vi "configureTimingNow.vi"(8 "error in (no error)":errorcluster, 11 "DIO64Output in":refnum<class "DIO64Output.lvclass">) -> (0 "error out":errorcluster, 3 "DIO64Output out":refnum<class "DIO64Output.lvclass">)   [LabVIEW 2009, in "Hardware.lvlib" / "Channels.lvlib" / "DIO64Output.lvclass"]
uses:
  DIO64Output.lvclass
  DIO64Output.lvclass/DIO64Output.ctl
  <userlib>/dio64_32.LLB/DIO64 attribute value.ctl
  <userlib>/dio64_32.LLB/DIO64 attribute id.ctl
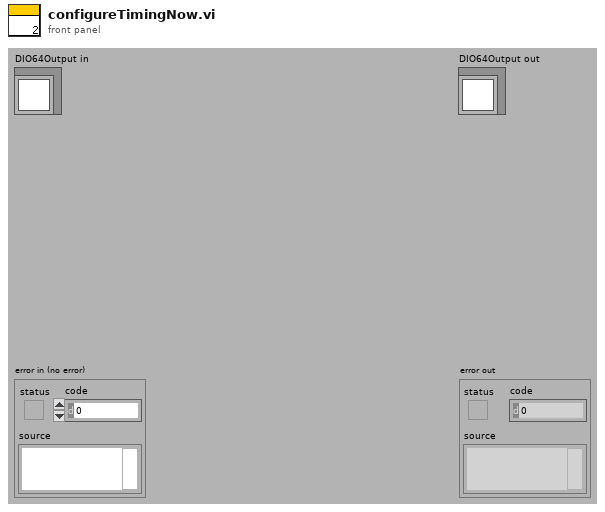
[diagram p1: front panel]
types:
  T1 = cluster{"Master Clock source":string, "Master Clock rate":dbl, "Start trigger line":string, "Scan rate":dbl, "Stop trigger line":string, "Sample Number":dbl}
  T2 = typedef "DIO64 Out Config Control.ctl" = cluster{"flags":enum16{"unused"}, "clock control":T3, "start trigger":T4, "stop trigger":T5, "DAQ clock modulo":u32, "repetitions":u32, "#transitions":u16}
  T3 = typedef "DIO64 clock control.ctl" = enum16{"internal", "external", "trig 0", "OCXO"}
  T4 = typedef "DIO64 start trig.ctl" = cluster{"source":enum16{"none", "internal", "external", "trig 2", "PXI Star"}, "type":enum16{"level", "edge", "edge to edge"}, "sense":enum16{"rising", "falling"}}
  T5 = typedef "DIO64 stop trig.ctl" = cluster{"source":enum16{"none", "internal", "external", "trig 3 in", "output FIFO"}, "type":enum16{"level", "edge"}, "sense":enum16{"falling", "rising"}}
  T6 = typedef "DIO64 attribute value.ctl" = enum16{"default", "long value", "polled", "interrupt", "packet", "demand", "local clock", "external clock", "rtsi/pxi clock", "precision clock", "20MHz", "10MHz", "precision OCXO", "enable", "disable"}
  T7 = typedef "DIO64 attribute id.ctl" = enum16{"input mode", "output mode", "input buffer size", "output buffer size", "major clock source", "input threshold percent", "output threshold percent", "input dma timeout", "rtsi/pxi global enable", "rtsi/pxi clock source", "rtsi clock/pxi trig 7 enable", "external clock enable", "pxi clock enable", "scan clock trig 0 enable", "start trig trig 2 enable", "stop trig trig 3 enable", "daq modulo trig 4 enable", "pxi star enable", "port routing", "staticOutputPorts", "serial number", "rearm enable", "SCLK enable", "FPGA info"}
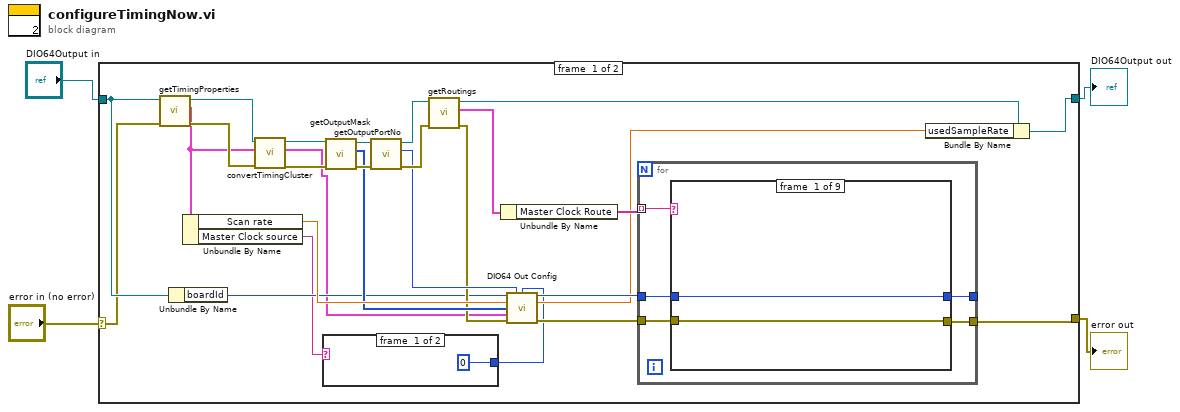
[diagram p0: block diagram]
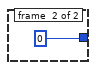
[diagram p2: hidden frame]
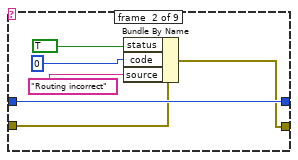
[diagram p3: hidden frame]
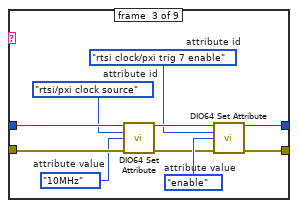
[diagram p4: hidden frame]
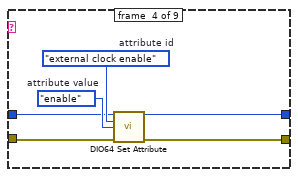
[diagram p5: hidden frame]
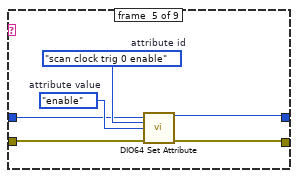
[diagram p6: hidden frame]
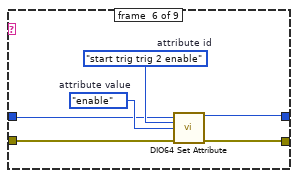
[diagram p7: hidden frame]
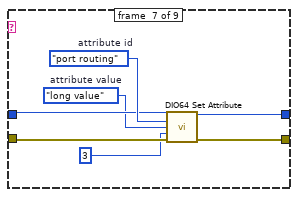
[diagram p8: hidden frame]
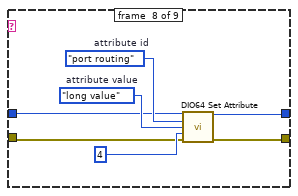
[diagram p9: hidden frame]
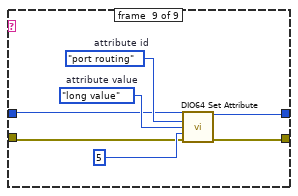
[diagram p10: hidden frame]
diagram:
  n1 = case shown="No Error" "error in (no error)" {
    selector: "error in (no error)" -> [w8 w96]
    tunnel: "DIO64Output in" -> [w10 w97]
    tunnel: [w12 w97] -> w2
    tunnel: [w22 w96] -> w1
    frame #0 {
      n2 = call-dynamic "getTimingProperties.vi"("error in (no error)"=w8, "DigitalOutput.lvclass in"=w10) -> ("error out"=w30:errorcluster, "Timing"=w17:T1, "DigitalOutput.lvclass out"=w31:refnum<class "DIO64Output.lvclass">)  [unwired: 7 in]
      n3 = Unbundle By Name(w10) -> ("boardId"=w9:i32)
      n4 = Unbundle By Name(w17) -> ("Scan rate"=w23:dbl, "Master Clock source"=w7:string)
      n5 = call "convertTimingCluster.vi"("error in (no error)"=w30, "Timing"=w17, "DIO64Output in"=w31) -> ("error out"=w26:errorcluster, "Out Config Control"=w5:T2, "DIO64Output out"=w27:refnum<class "DIO64Output.lvclass">)  [unwired: 6 in]
      n6 = case shown="\"PXI_Trig_00\"" w7 {
        tunnel: [u32 0 ("divider") 0] -> w6
        frame #0 {
        }
        frame #1 {
        }
      }
      n7 = call "getOutputMask.vi"("error in (no error)"=w26, "DIO64Output.lvclass in"=w27) -> ("error out"=w28:errorcluster, "mask"=w18:u16[], "DIO64Output.lvclass out"=w29:refnum<class "DIO64Output.lvclass">)  [unwired: 7 in]
      n8 = call "getOutputPortNo.vi"("error in (no error)"=w28, "DIO64Output.lvclass in"=w29) -> ("error out"=w24:errorcluster, "#ports"=w19:u8, "DIO64Output.lvclass out"=w25:refnum<class "DIO64Output.lvclass">)  [unwired: 7 in]
      n9 = call-dynamic "getRoutings.vi"("error in (no error)"=w24, "DigitalOutput.lvclass in"=w25) -> ("error out"=w14:errorcluster, "Routings"=w21:cluster{"Master Clock Route":string[]}, "DigitalOutput.lvclass out"=w13:refnum<class "DIO64Output.lvclass">)  [unwired: 7 in]
      n10 = Unbundle By Name(w21) -> ("Master Clock Route"=w20:string[])
      n11 = call <userlib>:"DIO64 Out Config.vi"("board in"=w9, "#ports"=w19, "divider"=w6, "scan rate (Hz)"=w23, "mask"=w18, "Config Control"=w5, "error in (no error)"=w14) -> ("board out"=w16:u16, "actual scan rate (Hz)"=w11:dbl, "error out"=w15:errorcluster)  [unwired: 6 in]
      n12 = for {
        tunnel: [w38] -> w22
        tunnel: w15 -> [w37]
        tunnel: w16 -> [w36]
        tunnel: [w35] -> _
        tunnel: w20 -> [w34] mode=indexing
        n13 = case shown="\"Dio64_10MHz to PXI_Trig_07\"" w34 {
          tunnel: [w39 w44 w47 w58 w63 w69 w78 w82 w90] -> w38
          tunnel: w37 -> [w39 w45 w55 w59 w65 w71 w79 w84 w91]
          tunnel: w36 -> [w40 w46 w56 w60 w66 w72 w80 w85 w92]
          tunnel: [w40 w46 w48 w57 w64 w70 w77 w83 w89] -> w35
          frame #0 {
          }
          frame #1 {
            n14 = Bundle By Name(cluster=w45, "status"=TRUE, "code"=0, "source"="Routing incorrect") -> (w44:errorcluster)
          }
          frame #2 {
            w50 = DIO64_attribute_value."enable"  # attribute value
            w51 = DIO64_attribute_id."rtsi clock/pxi trig 7 enable"  # attribute id
            w53 = DIO64_attribute_value."10MHz"  # attribute value
            w54 = DIO64_attribute_id."rtsi/pxi clock source"  # attribute id
            n15 = call <userlib>:"DIO64 Set Attribute.vi"("board in"=w56, "attribute id"=w54, "attribute value"=w53, "error in (no error)"=w55) -> ("board out"=w52:u16, "error out"=w49:errorcluster)  [unwired: 10 in]
            n16 = call <userlib>:"DIO64 Set Attribute.vi"("board in"=w52, "attribute id"=w51, "attribute value"=w50, "error in (no error)"=w49) -> ("board out"=w48:u16, "error out"=w47:errorcluster)  [unwired: 10 in]
          }
          frame #3 {
            w61 = DIO64_attribute_value."enable"  # attribute value
            w62 = DIO64_attribute_id."external clock enable"  # attribute id
            n17 = call <userlib>:"DIO64 Set Attribute.vi"("board in"=w60, "attribute id"=w62, "attribute value"=w61, "error in (no error)"=w59) -> ("board out"=w57:u16, "error out"=w58:errorcluster)  [unwired: 10 in]
          }
          frame #4 {
            w67 = DIO64_attribute_value."enable"  # attribute value
            w68 = DIO64_attribute_id."scan clock trig 0 enable"  # attribute id
            n18 = call <userlib>:"DIO64 Set Attribute.vi"("board in"=w66, "attribute id"=w68, "attribute value"=w67, "error in (no error)"=w65) -> ("board out"=w64:u16, "error out"=w63:errorcluster)  [unwired: 10 in]
          }
          frame #5 {
            w73 = DIO64_attribute_value."enable"  # attribute value
            w74 = DIO64_attribute_id."start trig trig 2 enable"  # attribute id
            n19 = call <userlib>:"DIO64 Set Attribute.vi"("board in"=w72, "attribute id"=w74, "attribute value"=w73, "error in (no error)"=w71) -> ("board out"=w70:u16, "error out"=w69:errorcluster)  [unwired: 10 in]
          }
          frame #6 {
            w76 = DIO64_attribute_value."long value"  # attribute value
            w81 = DIO64_attribute_id."port routing"  # attribute id
            n20 = call <userlib>:"DIO64 Set Attribute.vi"("board in"=w80, "attribute id"=w81, "attribute value"=w76, "value"=3, "error in (no error)"=w79) -> ("board out"=w77:u16, "error out"=w78:errorcluster)  [unwired: 9 in]
          }
          frame #7 {
            w87 = DIO64_attribute_value."long value"  # attribute value
            w86 = DIO64_attribute_id."port routing"  # attribute id
            n21 = call <userlib>:"DIO64 Set Attribute.vi"("board in"=w85, "attribute id"=w86, "attribute value"=w87, "value"=4, "error in (no error)"=w84) -> ("board out"=w83:u16, "error out"=w82:errorcluster)  [unwired: 9 in]
          }
          frame #8 {
            w94 = DIO64_attribute_value."long value"  # attribute value
            w93 = DIO64_attribute_id."port routing"  # attribute id
            n22 = call <userlib>:"DIO64 Set Attribute.vi"("board in"=w92, "attribute id"=w93, "attribute value"=w94, "value"=5, "error in (no error)"=w91) -> ("board out"=w89:u16, "error out"=w90:errorcluster)  [unwired: 9 in]
          }
        }
      }
      n23 = Bundle By Name(cluster=w13, "usedSampleRate"=w11) -> (w12:refnum<class "DIO64Output.lvclass">)
    }
    frame #1 {
    }
  }
  "error out" <- w1
  "DIO64Output out" <- w2
